vi "Launch_Create All Message Queues.vi"(8 "error in (no error)":errorcluster, 11 "This VI":refnum<vi>) -> (0 "error out":errorcluster, 3 "Message Queues out":T1)   [LabVIEW 2024, in "LaunchTest.lvlib" / "Launch_Message Queue.lvlib"]
doc: "This VI creates and initializes all the message queues for your application. If your application requires more than one message queue, right-click the \"Message Queues\" constant above and select Open Type Def. Add the new Message Queue(s) to the type definition, then initialize them in this VI."
uses:
  Launch_Message Queue.lvlib
  Launch_Message Cluster.ctl
  Launch_All Message Queues.ctl
  Launch_Enqueue Message (Single).vi
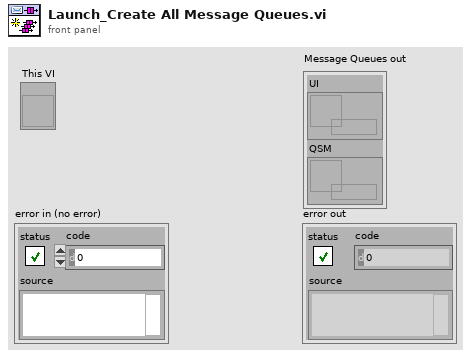
[diagram p1: front panel]
types:
  T1 = typedef "LaunchTest.lvlib/Launch_Message Queue.lvlib/Launch_All Message Queues.ctl" = cluster{"UI":refnum<queue>, "QSM":refnum<queue>}
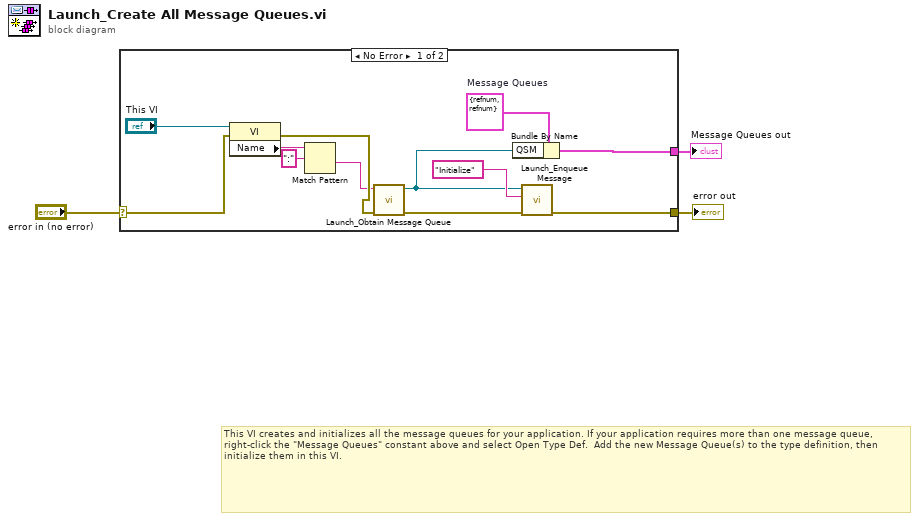
[diagram p0: block diagram]
diagram:
  # "This VI creates and initializes all the message queues for your application. If your application requires more than one message queue, right-click the \"Message Queues\" constant above and select Open Type Def.  Add the new Message Queue(s) to the type definition, then initialize them in this VI."
  n1 = case shown="No Error" "error in (no error)" {
    selector: "error in (no error)" -> [w7 w16]
    tunnel: [w15 w16] -> w3
    tunnel: [w13 _] -> w2
    frame No Error {
      w14 = T1 {"UI"=refnum, "QSM"=refnum}  # Message Queues
      n2 = property class="VI"(reference="This VI", error in=w7) -> (error out=w6:errorcluster, "Name"=w9:string)  [unwired: 1 out]
      n3 = Match Pattern(string=w9, regular expression=":") -> (after substring=w4:string)  [unwired: 1 in, 3 out]
      n4 = call "Launch_Obtain Message Queue.vi"("error in (no error)"=w6, "Queue Name"=w4) -> ("error out"=w12:errorcluster, "Message Queue"=w10:refnum<queue>)  [unwired: 8 in]
      n5 = Bundle By Name(cluster=w14, "QSM"=w10) -> (w13:T1)
      n6 = call-poly "Launch_Enqueue Message.vi"("error in (no error)"=w12, "Message"="Initialize", "Message Queue"=w10) -> ("error out"=w15:errorcluster)  [unwired: 7 in, 1 out]
    }
    frame Error {
    }
  }
  "Message Queues out" <- w2
  "error out" <- w3
